vi "WT300 Get Data.vi"(8 "error in (no error)":errorcluster, 11 "VISA resource name":refnum<visa-resource-name>) -> (0 "error out":errorcluster, 1 "Power":sgl caption="Measure Value" format="%.3f", 2 "VISA resource name out":refnum<visa-resource-name>, 3 "Power Data":T1={"Current (A):Element 1"=236.2, "Current (A):Element 2"=17.749, "Power (W):Sigma"=4192.0, "Watt Hours (Wh):Sigma"=0.0, "Voltage (V):Element 2"=236.2, "Voltage (V):Element 1"=236.2, "Current Crest Factor:Element 1"=0.0, "Current Crest Factor:Element 2"=0.0, "Voltage Harmonic (%):Element 1"=0.0, "Voltage Harmonic (%):Element 2"=0.0, "Voltage Crest Factor:Element 1"=0.0, "Voltage Crest Factor:Element 2"=0.0, "Time:Element 1"=0.0, "Frequency (Hz):Element 1"=0.0, "Apparent Power (VA):Element 1"=0.0, "Apparent Power (VA):Element 2"=0.0, "Power Factor:Element 1"=0.0, "Power Factor:Element 2"=0.0, "Max Watt Hours"=0.0, "Voltage (V):Element 2 Avg"=0.0, "Voltage (V):Element 1 Avg"=0.0} {"Voltage (V):Element 1 Avg" format="%.3g"; "Voltage (V):Element 2 Avg" format="%.3g"; "Max Watt Hours" format="%.3g"; "Power Factor:Element 2" format="%.3g"; "Power Factor:Element 1" format="%.3g"; "Apparent Power (VA):Element 2" format="%.3g"; "Apparent Power (VA):Element 1" format="%.3g"; "Frequency (Hz):Element 1" format="%.3g"; "Time:Element 1" format="%.3g"; "Voltage Crest Factor:Element 2" format="%.3g"; "Voltage Crest Factor:Element 1" format="%.3g"; "Voltage Harmonic (%):Element 2" format="%.3g"; "Voltage Harmonic (%):Element 1" format="%.3g"; "Current Crest Factor:Element 2" format="%.3g"; "Current Crest Factor:Element 1" format="%.3g"; "Voltage (V):Element 1" format="%.3g"; "Voltage (V):Element 2" format="%.3g"; "Watt Hours (Wh):Sigma" format="%.3f"; "Power (W):Sigma" format="%.3g"; "Current (A):Element 2" format="%.3g"; "Current (A):Element 1" format="%.3g"}, 5 "Yokogawa Data":string[][](array[string]), 7 "Yokogawa DBL Array":dbl[](array[numeric]))   [LabVIEW 2016]
uses:
  Trunk/Utility/Type Definitions/UTILITY Power Data.ctl
panel:
  in  "Dryer PowerData":T1={"Current (A):Element 1"=236.2, "Current (A):Element 2"=17.749, "Power (W):Sigma"=4192.0, "Watt Hours (Wh):Sigma"=0.0, "Voltage (V):Element 2"=236.2, "Voltage (V):Element 1"=236.2, "Current Crest Factor:Element 1"=0.0, "Current Crest Factor:Element 2"=0.0, "Voltage Harmonic (%):Element 1"=0.0, "Voltage Harmonic (%):Element 2"=0.0, "Voltage Crest Factor:Element 1"=0.0, "Voltage Crest Factor:Element 2"=0.0, "Time:Element 1"=0.0, "Frequency (Hz):Element 1"=0.0, "Apparent Power (VA):Element 1"=0.0, "Apparent Power (VA):Element 2"=0.0, "Power Factor:Element 1"=0.0, "Power Factor:Element 2"=0.0, "Max Watt Hours"=0.0, "Voltage (V):Element 2 Avg"=0.0, "Voltage (V):Element 1 Avg"=0.0} {"Voltage (V):Element 1 Avg" format="%.3g"; "Voltage (V):Element 2 Avg" format="%.3g"; "Max Watt Hours" format="%.3g"; "Power Factor:Element 2" format="%.3g"; "Power Factor:Element 1" format="%.3g"; "Apparent Power (VA):Element 2" format="%.3g"; "Apparent Power (VA):Element 1" format="%.3g"; "Frequency (Hz):Element 1" format="%.3g"; "Time:Element 1" format="%.3g"; "Voltage Crest Factor:Element 2" format="%.3g"; "Voltage Crest Factor:Element 1" format="%.3g"; "Voltage Harmonic (%):Element 2" format="%.3g"; "Voltage Harmonic (%):Element 1" format="%.3g"; "Current Crest Factor:Element 2" format="%.3g"; "Current Crest Factor:Element 1" format="%.3g"; "Voltage (V):Element 1" format="%.3g"; "Voltage (V):Element 2" format="%.3g"; "Watt Hours (Wh):Sigma" format="%.3f"; "Power (W):Sigma" format="%.3g"; "Current (A):Element 2" format="%.3g"; "Current (A):Element 1" format="%.3g"}
  # "Output Data from WT210"
  # "Wh"
  # "V"
  # "A"
  # "V Hz"
  # "W"
  # "PF"
  # "VA"
  # "V CF"
  # "A CF"
  # "WT210 can only take one harmonic reading"
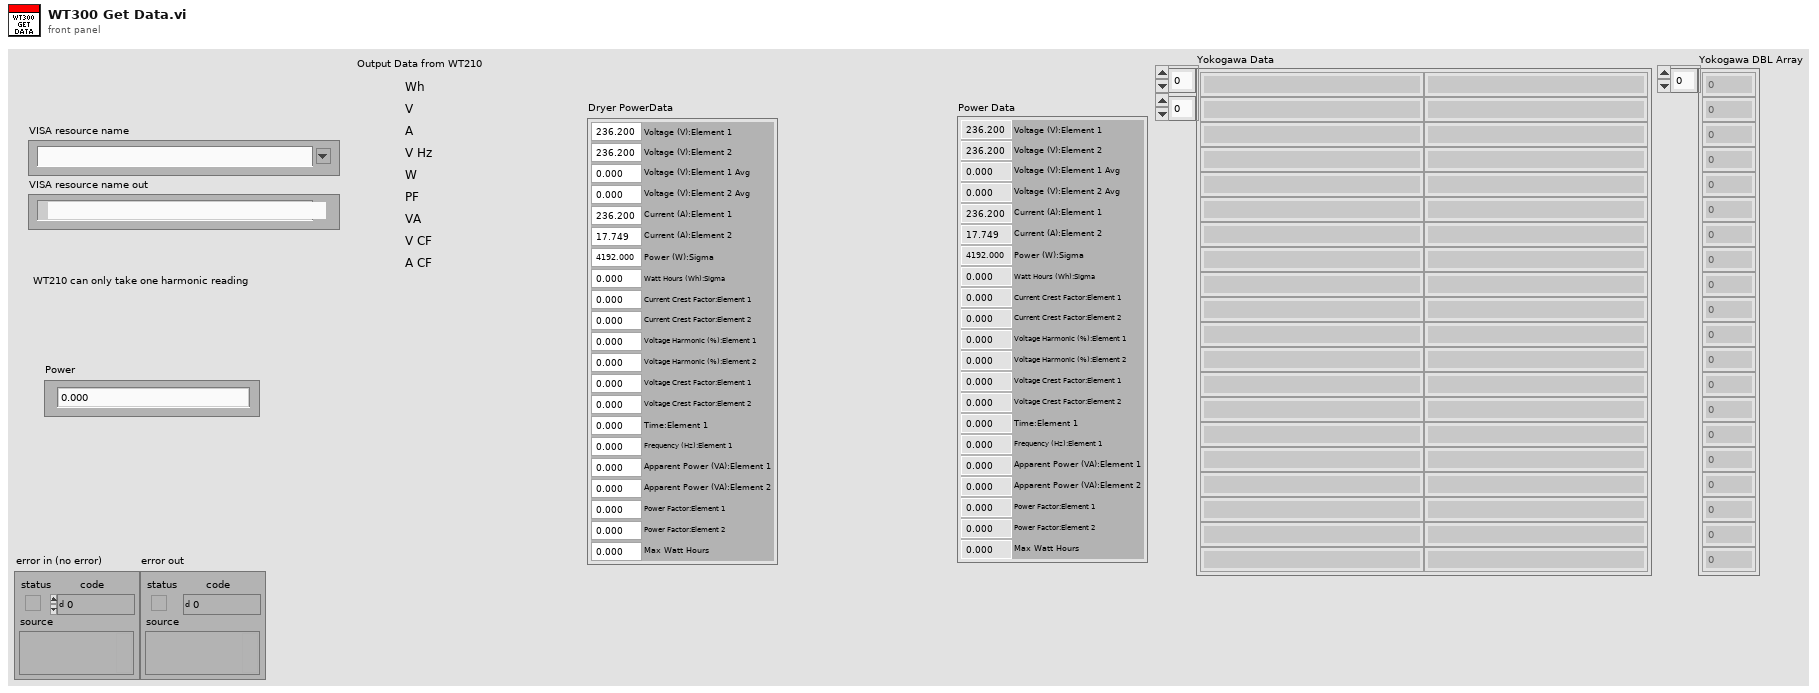
[diagram p1: front panel]
types:
  T1 = typedef "UTILITY Power Data.ctl" = cluster{"Current (A):Element 1":dbl, "Current (A):Element 2":dbl, "Power (W):Sigma":dbl, "Watt Hours (Wh):Sigma":dbl, "Voltage (V):Element 2":dbl, "Voltage (V):Element 1":dbl, "Current Crest Factor:Element 1":dbl, "Current Crest Factor:Element 2":dbl, "Voltage Harmonic (%):Element 1":dbl, "Voltage Harmonic (%):Element 2":dbl, "Voltage Crest Factor:Element 1":dbl, "Voltage Crest Factor:Element 2":dbl, "Time:Element 1":dbl, "Frequency (Hz):Element 1":dbl, "Apparent Power (VA):Element 1":dbl, "Apparent Power (VA):Element 2":dbl, "Power Factor:Element 1":dbl, "Power Factor:Element 2":dbl, "Max Watt Hours":dbl, "Voltage (V):Element 2 Avg":dbl, "Voltage (V):Element 1 Avg":dbl}
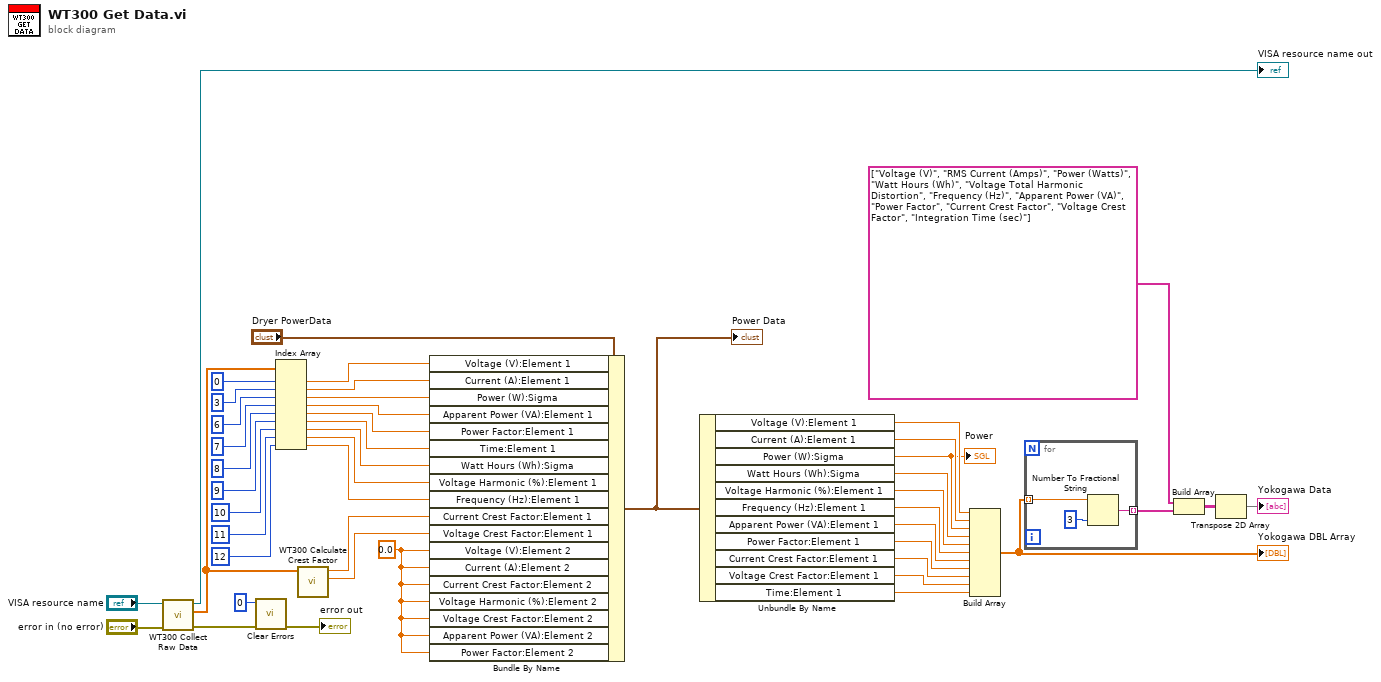
[diagram p0: block diagram]
diagram:
  w11 = 0.0 ("Urms:Element 2")
  n1 = call "WT300 Collect Raw Data.vi"("error in (no error)"="error in (no error)", "VISA Refnum in"="VISA resource name") -> ("error out"=w3:errorcluster, "Data"=w16:dbl[], "VISA resource name out"=→"VISA resource name out":refnum<visa-resource-name>)  [unwired: 6 in, 1 out]
  n2 = call <vilib>:"Clear Errors.vi"("error in (no error)"=w3, "specific error code to clear (0: all)"=0) -> ("error out"=→"error out":errorcluster)  [unwired: 4 in, 1 out]
  n3 = Index Array(array=w16, index #1=0 ("index"), index #2=3 ("index"), index #3=6 ("index"), index #4=7 ("index"), index #5=8 ("index"), index #6=9 ("index"), index #7=10 ("index"), index #8=11 ("index"), index #9=12 ("index")) -> (element #1=w27:dbl, element #2=w25:dbl, element #3=w23:dbl, element #4=w10:dbl, element #5=w9:dbl, element #6=w8:dbl, element #7=w18:dbl, element #8=w15:dbl, element #9=w13:dbl)
  n4 = call "WT300 Calculate Crest Factor.vi"("All Data"=w16) -> ("Voltage Crest Factor"=w6:dbl, "Current Crest Factor"=w7:dbl)  [unwired: 9 in]
  n5 = Bundle By Name(cluster="Dryer PowerData", "Voltage (V):Element 1"=w27, "Current (A):Element 1"=w25, "Power (W):Sigma"=w23, "Apparent Power (VA):Element 1"=w10, "Power Factor:Element 1"=w9, "Time:Element 1"=w8, "Watt Hours (Wh):Sigma"=w18, "Voltage Harmonic (%):Element 1"=w15, "Frequency (Hz):Element 1"=w13, "Current Crest Factor:Element 1"=w7, "Voltage Crest Factor:Element 1"=w6, "Voltage (V):Element 2"=w11, "Current (A):Element 2"=w11, "Current Crest Factor:Element 2"=w11, "Voltage Harmonic (%):Element 2"=w11, "Voltage Crest Factor:Element 2"=w11, "Apparent Power (VA):Element 2"=w11, "Power Factor:Element 2"=w11) -> (w44:T1)
  "Power Data" <- w44
  n6 = Unbundle By Name(w44) -> ("Voltage (V):Element 1"=w43:dbl, "Current (A):Element 1"=w42:dbl, "Power (W):Sigma"=w28:dbl, "Watt Hours (Wh):Sigma"=w41:dbl, "Voltage Harmonic (%):Element 1"=w40:dbl, "Frequency (Hz):Element 1"=w39:dbl, "Apparent Power (VA):Element 1"=w38:dbl, "Power Factor:Element 1"=w37:dbl, "Current Crest Factor:Element 1"=w36:dbl, "Voltage Crest Factor:Element 1"=w35:dbl, "Time:Element 1"=w30:dbl)
  "Power" <- w28
  n7 = Build Array(w43, w42, w28, w41, w40, w39, w38, w37, w36, w35, w30) -> (w32:dbl[])
  "Yokogawa DBL Array" <- w32
  n8 = for {
    tunnel: w32 -> [w48] mode=indexing
    tunnel: [w47] -> w5 mode=indexing
    n9 = Number To Fractional String(number=w48, precision (6)=i16 3) -> (F-format string=w47:string)  [unwired: 2 in]
  }
  n10 = Build Array(string[] ["Voltage (V)", "RMS Current (Amps)", "Power (Watts)", "Watt Hours (Wh)", "Voltage Total Harmonic Distortion", "Frequency (Hz)", "Apparent Power (VA)", "Power Factor", "Current Crest Factor", "Voltage Crest Factor", "Integration Time (sec)"], w5) -> (w4:string[][])
  n11 = Transpose 2D Array(2D array=w4) -> (transposed array=→"Yokogawa Data":string[][])
